vi "Moving Histogram PtByPt.vi"() -> ()   [LabVIEW 2023]
doc: "Calculates the histogram of a given signal as new data is acquired."
uses:
  <vilib>/ptbypt/NI_PtbyPt.lvlib
panel:
  in  "Reinitialize?":bool
  out "Vertical Histogram":T1(graph)
  out "Waveform Chart":dbl(graph)
  out "Histogram Graph":T2(graph)
  in  "Input signal":u16(ring) items=["Gaussian", "Sine", "Triangle"]
  in  "Stop":bool
  in  "Sample length":i32(slide)=1000 scale=10.0..2000.0
  in  "Number of intervals":i32(slide)=10 scale=5.0..20.0
  # "Overview: Calculates the histogram of a given signal and updates it as new data is acquired.\nRequirement: LabVIEW Full Development System\nInstructions:\n1. Run the VI.\n2. Choose the type of Input signal generated and observe the resulting histograms.\n3. Change the Number of intervals and Sample length and observe the effects on the histograms.\n4. Click Stop to stop the VI."
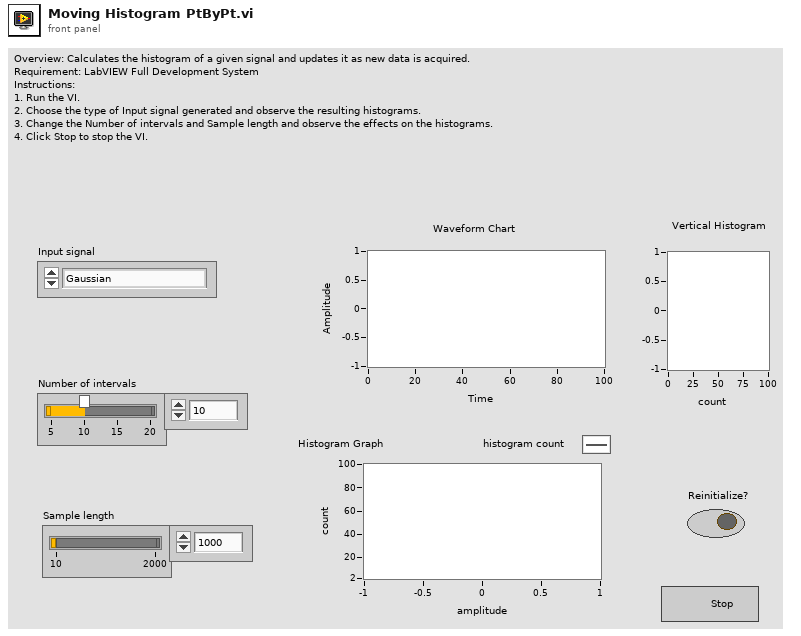
[diagram p1: front panel]
types:
  T1 = cluster{"Histogram: h(x)":i32[], "X Values":dbl[]}
  T2 = cluster{"X Values":dbl[], "Histogram: h(x)":i32[]}
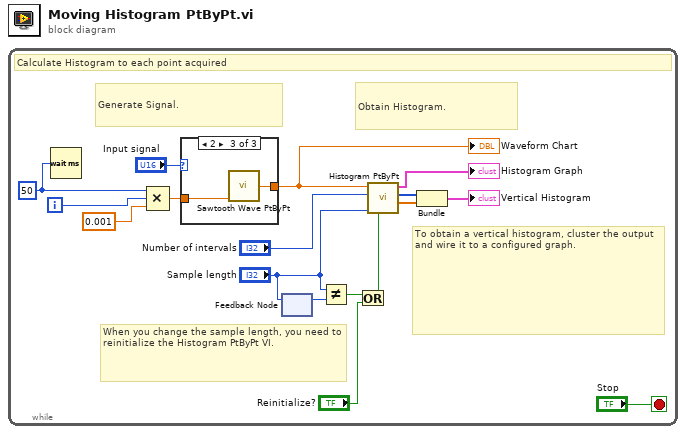
[diagram p0: block diagram]
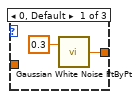
[diagram p2: hidden frame]
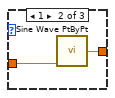
[diagram p3: hidden frame]
diagram:
  n1 = while {
    i -> [w2]
    stop <- "Stop" stop-if-true
    w3 = u32 50 ("milliseconds to wait")
    # "When you change the sample length, you need to reinitialize the Histogram PtByPt VI."
    # "To obtain a vertical histogram, cluster the output and wire it to a configured graph."
    # "Obtain Histogram."
    # "Generate Signal."
    # "Calculate Histogram to each point acquired"
    n2 = Wait (ms)(milliseconds to wait=w3) -> ()  [unwired: 1 out]
    n3 = Compound Arithmetic op=MULTIPLY(w3, w2, 0.001 ("y")) -> (w12:dbl)
    n4 = case shown="2" "Input signal" {
      tunnel: [w19 w21 w23] -> w13
      tunnel: w12 -> [_ w20 w22]
      frame 0, Default {
        n5 = call <vilib>:"Gaussian White Noise PtByPt.vi"("standard deviation"=0.3) -> ("Gaussian white noise"=w19:dbl)  [unwired: 2 in]
      }
      frame 1 {
        n6 = call <vilib>:"Sine Wave PtByPt.vi"("time"=w20) -> ("sine wave"=w21:dbl)  [unwired: 3 in]
      }
      frame 2 {
        n7 = call <vilib>:"Sawtooth Wave PtByPt.vi"("time"=w22) -> ("sawtooth wave"=w23:dbl)  [unwired: 3 in]
      }
    }
    "Waveform Chart" <- w13
    n8 = feedback-in #1("Sample length") -> ()
    n9 = feedback #1() -> (w7:i32)  [unwired: 1 in]
    n10 = Not Equal?(x="Sample length", y=w7) -> (x != y?=w6:bool)
    n11 = Or(x=w6, y="Reinitialize?") -> (x .or. y?=w5:bool)
    n12 = call <vilib>:"Histogram PtByPt.vi"("initialize"=w5, "sample length"="Sample length", "intervals"="Number of intervals", "x"=w13) -> ("X Values"=w10:dbl[], "Histogram: h(x)"=w11:i32[], "Histogram Graph"=→"Histogram Graph":T2)  [unwired: 5 out]
    n13 = Bundle("Histogram: h(x)"=w11, "X Values"=w10) -> (→"Vertical Histogram":T1)  [unwired: 1 in]
  }
